vi "OpenDatalogFileRef.vi"() -> (0 "error out":errorcluster, 2 "Created?":bool, 3 "tdms file out":refnum<k34>)   [LabVIEW 2014]
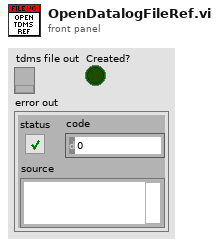
[diagram p1: front panel]
types:
  T1 = enum16{"open", "open or create", "create or replace", "create", "open (read-only)"}
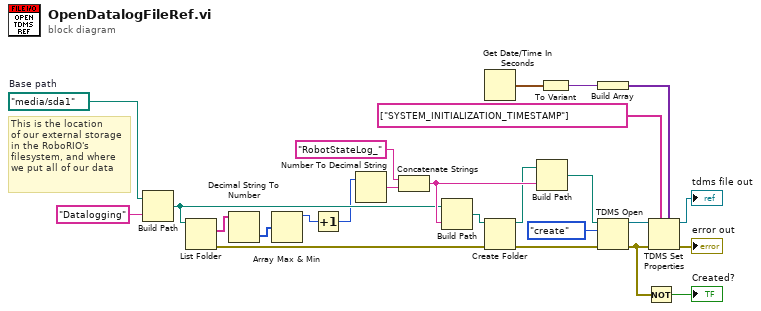
[diagram p0: block diagram]
diagram:
  w8 = path "/media/sda1"  # Base path
  # "This is the location\nof our external storage\nin the RoboRIO's\nfilesystem, and where\nwe put all of our data"
  n1 = Build Path(base path=w8, name or relative path="Datalogging") -> (appended path=w15:path)
  n2 = List Folder(path=w15) -> (filenames=w12:string[], error out=w5:errorcluster)  [unwired: 3 in, 2 out]
  n3 = Decimal String To Number(string=w12) -> (number=w7:i32[])  [unwired: 2 in, 1 out]
  n4 = Array Max & Min(array=w7) -> (max value=w6:i32)  [unwired: 3 out]
  n5 = Increment(x=w6) -> (x+1=w13:i32)
  n6 = Number To Decimal String(number=w13) -> (decimal integer string=w14:string)  [unwired: 1 in]
  n7 = Concatenate Strings("RobotStateLog_" ("string"), w14) -> (w19:string)
  n8 = Build Path(base path=w15, name or relative path=w19) -> (appended path=w17:path)
  n9 = Get Date/Time In Seconds() -> (seconds since 1Jan1904=w23:timestamp)
  n10 = Create Folder(path (use dialog)=w17, error in=w5) -> (created path=w18:path, error out=w4:errorcluster)  [unwired: 1 in, 1 out]
  n11 = Build Path(base path=w18, name or relative path=w19) -> (appended path=w20:path)
  n12 = To Variant(anything=w23) -> (Variant=w24:variant)
  n13 = Build Array(w24) -> (w25:variant[])
  n14 = TDMS Open(8:w4, 10:T1."create" ("operation (0:open)"), 11:w20) -> (0:w1:errorcluster, 3:w21:refnum<k34>)  [unwired: 4 in]
  n15 = Not(x=w1) -> (.not. x?=→"Created?":bool)
  n16 = TDMS Set Properties(5:w25, 7:string[] ["SYSTEM_INITIALIZATION_TIMESTAMP"] ("property names"), 8:w1, 11:w21) -> (0:→"error out":errorcluster, 3:→"tdms file out":refnum<k34>)  [unwired: 2 in, 2 out]
